vi "move_3.vi"(0 "Enum 3":enum16{"1", "2", "3", "4", "5"}(ring), 1 "Array 3":i32[](array[numeric]), 2 "Array 6":i32[](array[numeric]), 4 "Array in":i32[](array[numeric])) -> (5 "Array out":i32[](array[numeric]), 6 "Enum":T2(ring), 7 "Enum 2":T1(ring), 8 "Array 5":i32[](array[numeric]), 9 "Array 4":i32[](array[numeric]))   [LabVIEW 2016]
uses:
  <vilib>/NXT/Block Support/NXT_OutputPort.ctl
  <vilib>/NXT/NXTIO Xnodes/NXTIONodeSubVIs/NXTStopMotors.vi
  <vilib>/NXT/NXTIO Xnodes/NXTIONodeSubVIs/NXTMotorRunDistance.vi
  <vilib>/NXT/NXTIO Xnodes/NXTIONodeSubVIs/LEGOMotorStatus.vi
  <vilib>/NXT/NXTIO Xnodes/NXTIONodeSubVIs/NXTMoveMotors.vi
  <vilib>/NXT/NXTIO Xnodes/NXTIONodeSubVIs/LEGOResetMotors.vi
  <vilib>/NXT/Subs/LVHSConnector.ctl
  <vilib>/NXT/NXTIO Xnodes/AddressXNode/NXTIOAddress.xnode
  <vilib>/NXT/NXTIO Xnodes/NXTIOXNode/NXTIO.xnode
  <vilib>/NXT/LegoClasses/BrickReference/BrickReference.lvclass
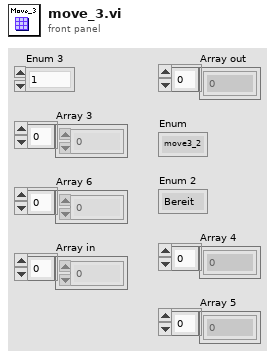
[diagram p1: front panel]
types:
  T1 = enum16{"Bereit", "Move 1", "Reference_pos", "Wait", "row1_check", "row2_check", "row3_check", "return", "move2", "move3", "move4", "move5", "end"}
  T2 = enum16{"move3_2", "move3_3", "move3_4", "move3_5"}
  T3 = enum16{"forward", "mark", "pause", "up", "return", "end"}
  T4 = typedef "NXT_OutputPort.ctl" = u8
  T5 = cluster{"Output Port":T4, "Output Port 2":T4, "Output Port 3":T4}
  T6 = enum16{"forward", "right", "mark", "pause", "up", "return", "end"}
  T7 = typedef "LVHSConnector.ctl" = refnum<class "BrickReference.lvclass">
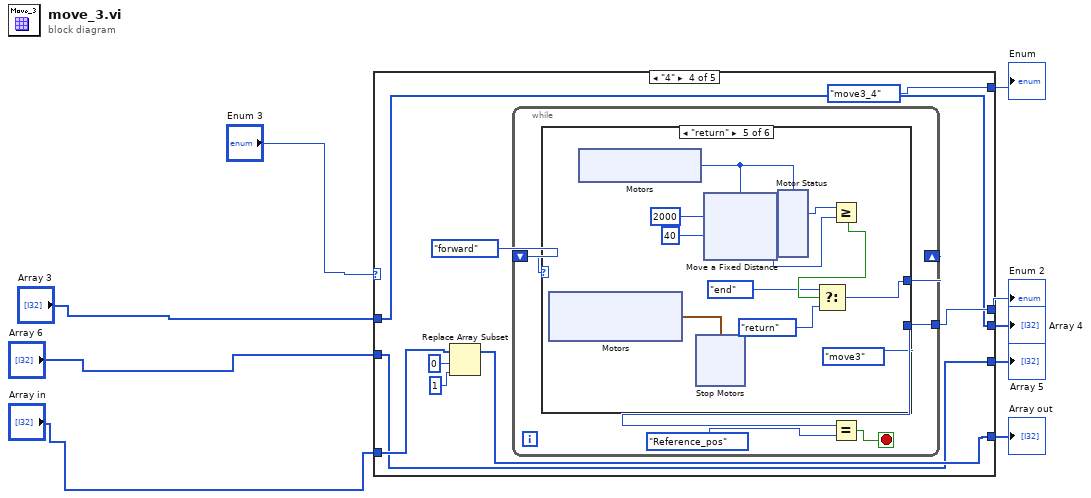
[diagram p0: block diagram]
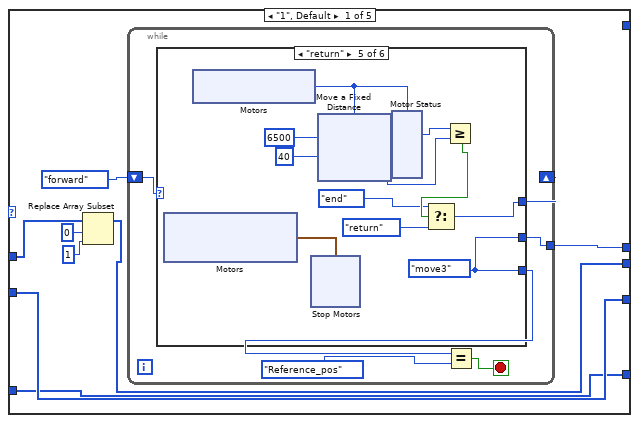
[diagram p2: hidden frame]
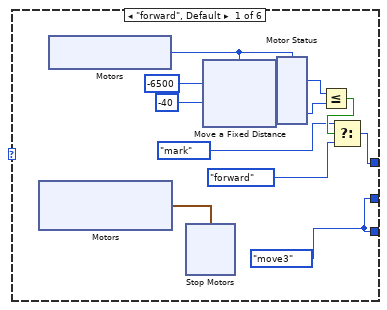
[diagram p3: hidden frame]
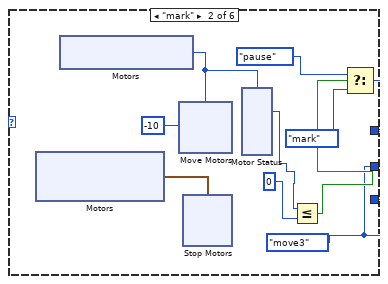
[diagram p4: hidden frame]
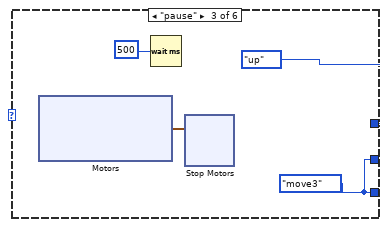
[diagram p5: hidden frame]
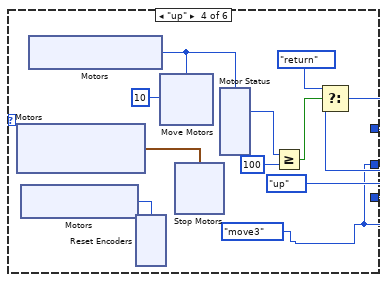
[diagram p6: hidden frame]
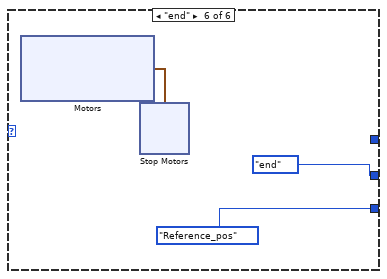
[diagram p7: hidden frame]
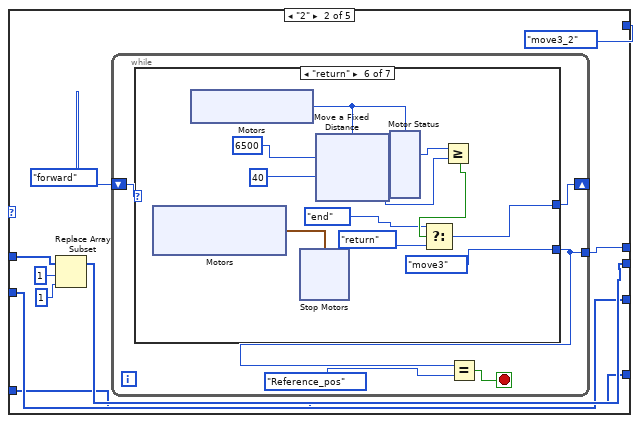
[diagram p8: hidden frame]
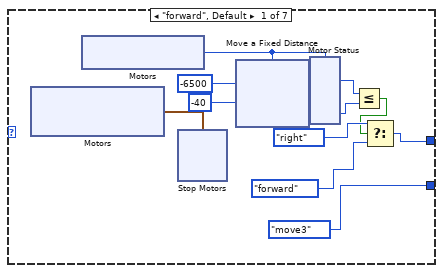
[diagram p9: hidden frame]
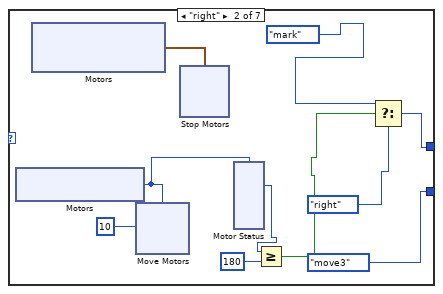
[diagram p10: hidden frame]
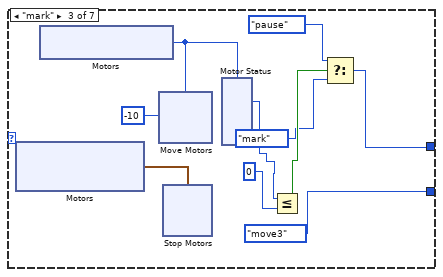
[diagram p11: hidden frame]
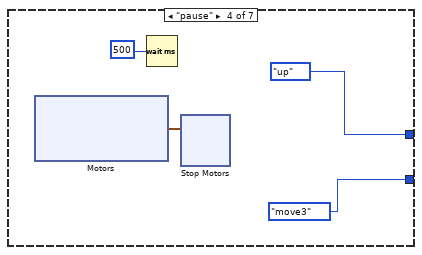
[diagram p12: hidden frame]
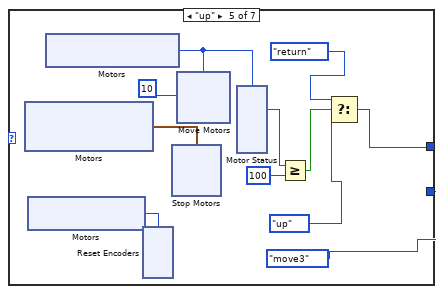
[diagram p13: hidden frame]
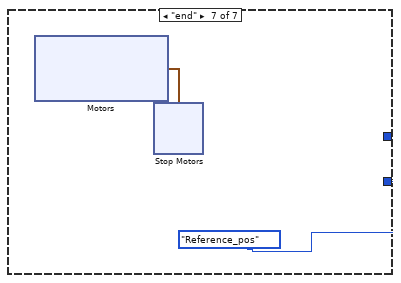
[diagram p14: hidden frame]
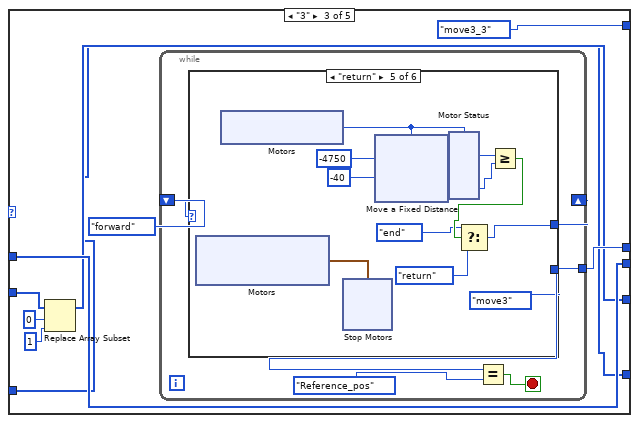
[diagram p15: hidden frame]
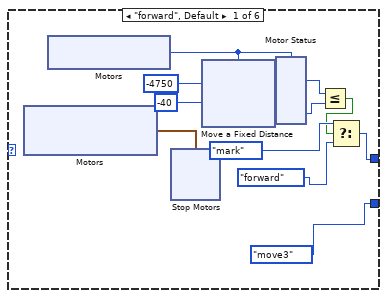
[diagram p16: hidden frame]
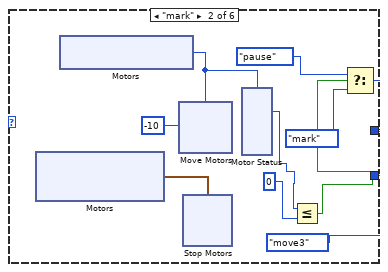
[diagram p17: hidden frame]
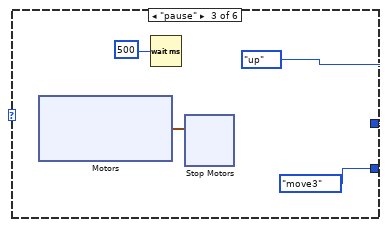
[diagram p18: hidden frame]
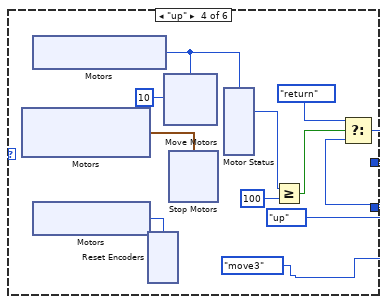
[diagram p19: hidden frame]
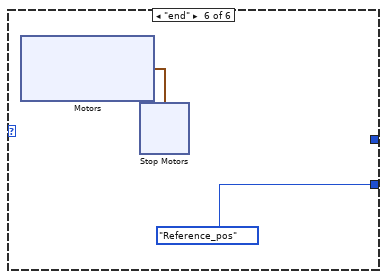
[diagram p20: hidden frame]
diagram:
  n1 = case shown="\"4\"" "Enum 3" {
    tunnel: [w16 w192 w398 w572 w745] -> w2
    tunnel: [_ T2."move3_2" T2."move3_3" T2."move3_4" T2."move3_5"] -> w3
    tunnel: "Array 6" -> [w15 w186 w393 w566 w738]
    tunnel: [w15 w186 w392 w566 w738] -> w5
    tunnel: [w10 w187 w396 w565 w739] -> w6
    tunnel: "Array 3" -> [w13 w188 w396 w565 w740]
    tunnel: [w14 w185 w391 w567 w741] -> w8
    tunnel: "Array in" -> [w14 w185 w391 w568 w741]
    frame "1", Default {
      n2 = Replace Array Subset(array=w13, new element=1 ("new element/subarray"), index=0) -> (w10:i32[])
      n3 = while {
        shift-right: [w23] -> _
        shift-left: T3."forward" -> [w22]
        tunnel: [w18] -> w16
        stop <- w20 stop-if-true
        n4 = case shown="\"return\"" w22 {
          tunnel: [w24 w67 T3."up" w109 w140 _] -> w23
          tunnel: [w33 w60 w92 w103 w149 T1."Reference_pos"] -> w21
          tunnel: [w33 w60 w92 w103 w149 T1."end"] -> w18
          frame "forward", Default {
            w28 = -6500 ("Distance 1")
            w33 = T1."move3"
            n5 = xnode "Motors"() -> ("Motor"=w34:cluster{"Port":T4, "Port":T4})
            n6 = xnode "Motors"() -> ("Motor"=w30:T4)
            n7 = xnode "Stop Motors"("Motors"=w34) -> ()  [unwired: 1 in, 1 out]
            n8 = xnode "Move a Fixed Distance"("Speed 1"=i8 -40, "Distance 1"=w28, "Motors"=w30) -> ("NXT/EV3"=w29:T7)  [unwired: 1 in]
            n9 = xnode "Motor Status"("Motors"=w30, "NXT/EV3"=w29) -> ("Position 1"=w31:i32)  [unwired: 2 out]
            n10 = Less Or Equal?(x=w31, y=w28) -> (x <= y?=w27:bool)
            n11 = Select(t=T3."mark", s=w27, f=T3."forward") -> (s? t:f=w24:T3)
          }
          frame "mark" {
            w60 = T1."move3"
            n12 = xnode "Motors"() -> ("Motor"=w69:cluster{"Port":T4, "Port":T4})
            n13 = xnode "Motors"() -> ("Motor"=w64:T4)
            n14 = xnode "Move Motors"("Power/Speed 1"=i8 -10, "Motors"=w64) -> ()  [unwired: 1 in, 1 out]
            n15 = xnode "Stop Motors"("Motors"=w69) -> ()  [unwired: 1 in, 1 out]
            n16 = xnode "Motor Status"("Motors"=w64) -> ("Position 1"=w63:i32)  [unwired: 1 in, 2 out]
            n17 = Less Or Equal?(x=w63, y=0) -> (x <= y?=w61:bool)
            n18 = Select(t=T3."pause", s=w61, f=T3."mark") -> (s? t:f=w67:T3)
          }
          frame "pause" {
            w92 = T1."move3"
            n19 = xnode "Motors"() -> ("Motor"=w95:cluster{"Port":T4, "Port":T4, "Port":T4})
            n20 = Wait (ms)(milliseconds to wait=u32 500 ("millisecond timer value")) -> ()  [unwired: 1 out]
            n21 = xnode "Stop Motors"("Motors"=w95) -> ()  [unwired: 1 in, 1 out]
          }
          frame "up" {
            w103 = T1."move3"
            n22 = xnode "Motors"() -> ("Motor"=w111:cluster{"Port":T4, "Port":T4})
            n23 = xnode "Motors"() -> ("Motor"=w102:T4)
            n24 = xnode "Motors"() -> ("Motor"=w105:T4)
            n25 = xnode "Reset Encoders"("Motors"=w102) -> ()  [unwired: 1 in, 1 out]
            n26 = xnode "Move Motors"("Power/Speed 1"=i8 10, "Motors"=w105) -> ()  [unwired: 1 in, 1 out]
            n27 = xnode "Stop Motors"("Motors"=w111) -> ()  [unwired: 1 in, 1 out]
            n28 = xnode "Motor Status"("Motors"=w105) -> ("Position 1"=w106:i32)  [unwired: 1 in, 2 out]
            n29 = Greater Or Equal?(x=w106, y=100) -> (x >= y?=w110:bool)
            n30 = Select(t=T3."return", s=w110, f=T3."up") -> (s? t:f=w109:T3)
          }
          frame "return" {
            w144 = 6500 ("Distance 1")
            w149 = T1."move3"
            n31 = xnode "Motors"() -> ("Motor"=w150:cluster{"Port":T4, "Port":T4})
            n32 = xnode "Motors"() -> ("Motor"=w147:T4)
            n33 = xnode "Stop Motors"("Motors"=w150) -> ()  [unwired: 1 in, 1 out]
            n34 = xnode "Move a Fixed Distance"("Speed 1"=i8 40, "Distance 1"=w144, "Motors"=w147) -> ("NXT/EV3"=w146:T7)  [unwired: 1 in]
            n35 = xnode "Motor Status"("Motors"=w147, "NXT/EV3"=w146) -> ("Position 1"=w145:i32)  [unwired: 2 out]
            n36 = Greater Or Equal?(x=w145, y=w144) -> (x >= y?=w143:bool)
            n37 = Select(t=T3."end", s=w143, f=T3."return") -> (s? t:f=w140:T3)
          }
          frame "end" {
            n38 = xnode "Motors"() -> ("Motor"=w178:cluster{"Port":T4, "Port":T4, "Port":T4})
            n39 = xnode "Stop Motors"("Motors"=w178) -> ()  [unwired: 1 in, 1 out]
          }
        }
        n40 = Equal?(x=w21, y=T1."Reference_pos") -> (x = y?=w20:bool)
      }
    }
    frame "2" {
      n41 = Replace Array Subset(array=w188, new element=1 ("new element/subarray"), index=1) -> (w187:i32[])
      n42 = while {
        shift-right: [w194] -> _
        shift-left: T6."forward" -> [w195]
        tunnel: [w198] -> w192
        stop <- w197 stop-if-true
        n43 = case shown="\"return\"" w195 {
          tunnel: [w200 w236 w268 T6."up" w310 w347 _] -> w194
          tunnel: [T1."move3" T1."move3" T1."move3" T1."move3" T1."move3" T1."move3" T1."Reference_pos"] -> w198
          frame "forward", Default {
            w203 = -6500 ("Distance 1")
            n44 = xnode "Motors"() -> ("Motor"=w209:cluster{"Port":T4, "Port":T4})
            n45 = xnode "Motors"() -> ("Motor"=w205:T4)
            n46 = xnode "Stop Motors"("Motors"=w209) -> ()  [unwired: 1 in, 1 out]
            n47 = xnode "Move a Fixed Distance"("Speed 1"=i8 -40, "Distance 1"=w203, "Motors"=w205) -> ("NXT/EV3"=w204:T7)  [unwired: 1 in]
            n48 = xnode "Motor Status"("Motors"=w205, "NXT/EV3"=w204) -> ("Position 1"=w206:i32)  [unwired: 2 out]
            n49 = Less Or Equal?(x=w206, y=w203) -> (x <= y?=w199:bool)
            n50 = Select(t=T6."right", s=w199, f=T6."forward") -> (s? t:f=w200:T6)
          }
          frame "right" {
            n51 = xnode "Motors"() -> ("Motor"=w244:T4)
            n52 = xnode "Motors"() -> ("Motor"=w243:cluster{"Port":T4, "Port":T4})
            n53 = xnode "Move Motors"("Power/Speed 1"=i8 10, "Motors"=w244) -> ()  [unwired: 1 in, 1 out]
            n54 = xnode "Stop Motors"("Motors"=w243) -> ()  [unwired: 1 in, 1 out]
            n55 = xnode "Motor Status"("Motors"=w244) -> ("Position 1"=w241:i32)  [unwired: 1 in, 2 out]
            n56 = Greater Or Equal?(x=w241, y=180) -> (x >= y?=w240:bool)
            n57 = Select(t=T6."mark", s=w240, f=T6."right") -> (s? t:f=w236:T6)
          }
          frame "mark" {
            n58 = xnode "Motors"() -> ("Motor"=w276:cluster{"Port":T4, "Port":T4})
            n59 = xnode "Motors"() -> ("Motor"=w274:T4)
            n60 = xnode "Move Motors"("Power/Speed 1"=i8 -10, "Motors"=w274) -> ()  [unwired: 1 in, 1 out]
            n61 = xnode "Stop Motors"("Motors"=w276) -> ()  [unwired: 1 in, 1 out]
            n62 = xnode "Motor Status"("Motors"=w274) -> ("Position 1"=w273:i32)  [unwired: 1 in, 2 out]
            n63 = Less Or Equal?(x=w273, y=0) -> (x <= y?=w271:bool)
            n64 = Select(t=T6."pause", s=w271, f=T6."mark") -> (s? t:f=w268:T6)
          }
          frame "pause" {
            n65 = xnode "Motors"() -> ("Motor"=w302:cluster{"Port":T4, "Port":T4, "Port":T4})
            n66 = Wait (ms)(milliseconds to wait=u32 500 ("millisecond timer value")) -> ()  [unwired: 1 out]
            n67 = xnode "Stop Motors"("Motors"=w302) -> ()  [unwired: 1 in, 1 out]
          }
          frame "up" {
            n68 = xnode "Motors"() -> ("Motor"=w317:cluster{"Port":T4, "Port":T4})
            n69 = xnode "Motors"() -> ("Motor"=w309:T4)
            n70 = xnode "Motors"() -> ("Motor"=w314:T4)
            n71 = xnode "Reset Encoders"("Motors"=w309) -> ()  [unwired: 1 in, 1 out]
            n72 = xnode "Stop Motors"("Motors"=w317) -> ()  [unwired: 1 in, 1 out]
            n73 = xnode "Move Motors"("Power/Speed 1"=i8 10, "Motors"=w314) -> ()  [unwired: 1 in, 1 out]
            n74 = xnode "Motor Status"("Motors"=w314) -> ("Position 1"=w315:i32)  [unwired: 1 in, 2 out]
            n75 = Greater Or Equal?(x=w315, y=100) -> (x >= y?=w316:bool)
            n76 = Select(t=T6."return", s=w316, f=T6."up") -> (s? t:f=w310:T6)
          }
          frame "return" {
            w351 = 6500 ("Distance 1")
            n77 = xnode "Motors"() -> ("Motor"=w356:cluster{"Port":T4, "Port":T4})
            n78 = xnode "Motors"() -> ("Motor"=w355:T4)
            n79 = xnode "Stop Motors"("Motors"=w356) -> ()  [unwired: 1 in, 1 out]
            n80 = xnode "Move a Fixed Distance"("Speed 1"=i8 40, "Distance 1"=w351, "Motors"=w355) -> ("NXT/EV3"=w354:T7)  [unwired: 1 in]
            n81 = xnode "Motor Status"("Motors"=w355, "NXT/EV3"=w354) -> ("Position 1"=w353:i32)  [unwired: 2 out]
            n82 = Greater Or Equal?(x=w353, y=w351) -> (x >= y?=w352:bool)
            n83 = Select(t=T6."end", s=w352, f=T6."return") -> (s? t:f=w347:T6)
          }
          frame "end" {
            n84 = xnode "Motors"() -> ("Motor"=w383:cluster{"Port":T4, "Port":T4, "Port":T4})
            n85 = xnode "Stop Motors"("Motors"=w383) -> ()  [unwired: 1 in, 1 out]
          }
        }
        n86 = Equal?(x=w198, y=T1."Reference_pos") -> (x = y?=w197:bool)
      }
    }
    frame "3" {
      n87 = Replace Array Subset(array=w393, new element=1 ("new element/subarray"), index=0) -> (w392:i32[])
      n88 = while {
        shift-right: [w404] -> _
        shift-left: T3."forward" -> [w403]
        tunnel: [w402] -> w398
        stop <- w401 stop-if-true
        n89 = case shown="\"return\"" w403 {
          tunnel: [w405 w448 T3."up" w490 w521 _] -> w404
          tunnel: [T1."move3" T1."move3" T1."move3" T1."move3" T1."move3" T1."Reference_pos"] -> w402
          frame "forward", Default {
            w409 = -4750 ("Distance 1")
            n90 = xnode "Motors"() -> ("Motor"=w415:cluster{"Port":T4, "Port":T4})
            n91 = xnode "Motors"() -> ("Motor"=w411:T4)
            n92 = xnode "Stop Motors"("Motors"=w415) -> ()  [unwired: 1 in, 1 out]
            n93 = xnode "Move a Fixed Distance"("Speed 1"=i8 -40, "Distance 1"=w409, "Motors"=w411) -> ("NXT/EV3"=w410:T7)  [unwired: 1 in]
            n94 = xnode "Motor Status"("Motors"=w411, "NXT/EV3"=w410) -> ("Position 1"=w412:i32)  [unwired: 2 out]
            n95 = Less Or Equal?(x=w412, y=w409) -> (x <= y?=w406:bool)
            n96 = Select(t=T3."mark", s=w406, f=T3."forward") -> (s? t:f=w405:T3)
          }
          frame "mark" {
            n97 = xnode "Motors"() -> ("Motor"=w450:cluster{"Port":T4, "Port":T4})
            n98 = xnode "Motors"() -> ("Motor"=w445:T4)
            n99 = xnode "Move Motors"("Power/Speed 1"=i8 -10, "Motors"=w445) -> ()  [unwired: 1 in, 1 out]
            n100 = xnode "Stop Motors"("Motors"=w450) -> ()  [unwired: 1 in, 1 out]
            n101 = xnode "Motor Status"("Motors"=w445) -> ("Position 1"=w444:i32)  [unwired: 1 in, 2 out]
            n102 = Less Or Equal?(x=w444, y=0) -> (x <= y?=w442:bool)
            n103 = Select(t=T3."pause", s=w442, f=T3."mark") -> (s? t:f=w448:T3)
          }
          frame "pause" {
            n104 = xnode "Motors"() -> ("Motor"=w476:cluster{"Port":T4, "Port":T4, "Port":T4})
            n105 = Wait (ms)(milliseconds to wait=u32 500 ("millisecond timer value")) -> ()  [unwired: 1 out]
            n106 = xnode "Stop Motors"("Motors"=w476) -> ()  [unwired: 1 in, 1 out]
          }
          frame "up" {
            n107 = xnode "Motors"() -> ("Motor"=w492:cluster{"Port":T4, "Port":T4})
            n108 = xnode "Motors"() -> ("Motor"=w486:T4)
            n109 = xnode "Motors"() -> ("Motor"=w483:T4)
            n110 = xnode "Reset Encoders"("Motors"=w483) -> ()  [unwired: 1 in, 1 out]
            n111 = xnode "Move Motors"("Power/Speed 1"=i8 10, "Motors"=w486) -> ()  [unwired: 1 in, 1 out]
            n112 = xnode "Stop Motors"("Motors"=w492) -> ()  [unwired: 1 in, 1 out]
            n113 = xnode "Motor Status"("Motors"=w486) -> ("Position 1"=w487:i32)  [unwired: 1 in, 2 out]
            n114 = Greater Or Equal?(x=w487, y=100) -> (x >= y?=w491:bool)
            n115 = Select(t=T3."return", s=w491, f=T3."up") -> (s? t:f=w490:T3)
          }
          frame "return" {
            w525 = -4750 ("Distance 1")
            n116 = xnode "Motors"() -> ("Motor"=w531:cluster{"Port":T4, "Port":T4})
            n117 = xnode "Motors"() -> ("Motor"=w528:T4)
            n118 = xnode "Stop Motors"("Motors"=w531) -> ()  [unwired: 1 in, 1 out]
            n119 = xnode "Move a Fixed Distance"("Speed 1"=i8 -40, "Distance 1"=w525, "Motors"=w528) -> ("NXT/EV3"=w527:T7)  [unwired: 1 in]
            n120 = xnode "Motor Status"("Motors"=w528, "NXT/EV3"=w527) -> ("Position 1"=w526:i32)  [unwired: 2 out]
            n121 = Greater Or Equal?(x=w526, y=w525) -> (x >= y?=w524:bool)
            n122 = Select(t=T3."end", s=w524, f=T3."return") -> (s? t:f=w521:T3)
          }
          frame "end" {
            n123 = xnode "Motors"() -> ("Motor"=w558:cluster{"Port":T4, "Port":T4, "Port":T4})
            n124 = xnode "Stop Motors"("Motors"=w558) -> ()  [unwired: 1 in, 1 out]
          }
        }
        n125 = Equal?(x=w402, y=T1."Reference_pos") -> (x = y?=w401:bool)
      }
    }
    frame "4" {
      n126 = Replace Array Subset(array=w568, new element=1 ("new element/subarray"), index=0) -> (w567:i32[])
      n127 = while {
        shift-right: [w578] -> _
        shift-left: T3."forward" -> [w577]
        tunnel: [w576] -> w572
        stop <- w575 stop-if-true
        n128 = case shown="\"return\"" w577 {
          tunnel: [w580 w622 w647 w663 w695 _] -> w578
          tunnel: [T1."move3" T1."move3" T1."move3" T1."move3" T1."move3" T1."Reference_pos"] -> w576
          frame "forward", Default {
            w583 = -3000 ("Distance 1")
            n129 = xnode "Motors"() -> ("Motor"=w585:T4)
            n130 = xnode "Motors"() -> ("Motor"=w589:cluster{"Port":T4, "Port":T4})
            n131 = xnode "Stop Motors"("Motors"=w589) -> ()  [unwired: 1 in, 1 out]
            n132 = xnode "Move a Fixed Distance"("Speed 1"=i8 -40, "Distance 1"=w583, "Motors"=w585) -> ("NXT/EV3"=w584:T7)  [unwired: 1 in]
            n133 = xnode "Motor Status"("Motors"=w585, "NXT/EV3"=w584) -> ("Position 1"=w586:i32)  [unwired: 2 out]
            n134 = Less Or Equal?(x=w586, y=w583) -> (x <= y?=w579:bool)
            n135 = Select(t=T3."mark", s=w579, f=T3."forward") -> (s? t:f=w580:T3)
          }
          frame "mark" {
            n136 = xnode "Motors"() -> ("Motor"=w624:cluster{"Port":T4, "Port":T4})
            n137 = xnode "Motors"() -> ("Motor"=w619:T4)
            n138 = xnode "Move Motors"("Power/Speed 1"=i8 -10, "Motors"=w619) -> ()  [unwired: 1 in, 1 out]
            n139 = xnode "Stop Motors"("Motors"=w624) -> ()  [unwired: 1 in, 1 out]
            n140 = xnode "Motor Status"("Motors"=w619) -> ("Position 1"=w618:i32)  [unwired: 1 in, 2 out]
            n141 = Less Or Equal?(x=w618, y=0) -> (x <= y?=w616:bool)
            n142 = Select(t=T3."pause", s=w616, f=T3."mark") -> (s? t:f=w622:T3)
          }
          frame "pause" {
            n143 = xnode "Motors"() -> ("Motor"=w648:cluster{"Port":T4, "Port":T4})
            n144 = call "x0_move2.vi"() -> ("Enum"=w647:T3)  [unwired: 1 in]
            n145 = xnode "Stop Motors"("Motors"=w648) -> ()  [unwired: 1 in, 1 out]
          }
          frame "up" {
            n146 = xnode "Motors"() -> ("Motor"=w665:cluster{"Port":T4, "Port":T4})
            n147 = xnode "Motors"() -> ("Motor"=w656:T4)
            n148 = xnode "Motors"() -> ("Motor"=w659:T4)
            n149 = xnode "Reset Encoders"("Motors"=w656) -> ()  [unwired: 1 in, 1 out]
            n150 = xnode "Stop Motors"("Motors"=w665) -> ()  [unwired: 1 in, 1 out]
            n151 = xnode "Move Motors"("Power/Speed 1"=i8 10, "Motors"=w659) -> ()  [unwired: 1 in, 1 out]
            n152 = xnode "Motor Status"("Motors"=w659) -> ("Position 1"=w660:i32)  [unwired: 1 in, 2 out]
            n153 = Greater Or Equal?(x=w660, y=100) -> (x >= y?=w664:bool)
            n154 = Select(t=T3."return", s=w664, f=T3."up") -> (s? t:f=w663:T3)
          }
          frame "return" {
            w694 = 2000 ("Distance 1")
            n155 = xnode "Motors"() -> ("Motor"=w704:cluster{"Port":T4, "Port":T4})
            n156 = xnode "Motors"() -> ("Motor"=w701:T4)
            n157 = xnode "Stop Motors"("Motors"=w704) -> ()  [unwired: 1 in, 1 out]
            n158 = xnode "Move a Fixed Distance"("Speed 1"=i8 40, "Distance 1"=w694, "Motors"=w701) -> ("NXT/EV3"=w700:T7)  [unwired: 1 in]
            n159 = xnode "Motor Status"("Motors"=w701, "NXT/EV3"=w700) -> ("Position 1"=w699:i32)  [unwired: 2 out]
            n160 = Greater Or Equal?(x=w699, y=w694) -> (x >= y?=w698:bool)
            n161 = Select(t=T3."end", s=w698, f=T3."return") -> (s? t:f=w695:T3)
          }
          frame "end" {
            n162 = xnode "Motors"() -> ("Motor"=w731:cluster{"Port":T4, "Port":T4, "Port":T4})
            n163 = xnode "Stop Motors"("Motors"=w731) -> ()  [unwired: 1 in, 1 out]
          }
        }
        n164 = Equal?(x=w576, y=T1."Reference_pos") -> (x = y?=w575:bool)
      }
    }
    frame "5" {
      n165 = Replace Array Subset(array=w740, new element=1 ("new element/subarray"), index=2) -> (w739:i32[])
      n166 = while {
        shift-right: [w747] -> _
        shift-left: T6."forward" -> [w748]
        tunnel: [w751] -> w745
        stop <- w750 stop-if-true
        n167 = case shown="\"return\"" w748 {
          tunnel: [w754 w789 w821 T6."up" w863 w900 _] -> w747
          tunnel: [T1."move3" T1."move3" T1."move3" T1."move3" T1."move3" T1."move3" T1."Reference_pos"] -> w751
          frame "forward", Default {
            w756 = -6500 ("Distance 1")
            n168 = xnode "Motors"() -> ("Motor"=w758:T4)
            n169 = xnode "Motors"() -> ("Motor"=w762:cluster{"Port":T4, "Port":T4})
            n170 = xnode "Move a Fixed Distance"("Speed 1"=i8 -40, "Distance 1"=w756, "Motors"=w758) -> ("NXT/EV3"=w757:T7)  [unwired: 1 in]
            n171 = xnode "Stop Motors"("Motors"=w762) -> ()  [unwired: 1 in, 1 out]
            n172 = xnode "Motor Status"("Motors"=w758, "NXT/EV3"=w757) -> ("Position 1"=w759:i32)  [unwired: 2 out]
            n173 = Less Or Equal?(x=w759, y=w756) -> (x <= y?=w755:bool)
            n174 = Select(t=T6."right", s=w755, f=T6."forward") -> (s? t:f=w754:T6)
          }
          frame "right" {
            n175 = xnode "Motors"() -> ("Motor"=w797:T4)
            n176 = xnode "Motors"() -> ("Motor"=w796:cluster{"Port":T4, "Port":T4})
            n177 = xnode "Move Motors"("Power/Speed 1"=i8 10, "Motors"=w797) -> ()  [unwired: 1 in, 1 out]
            n178 = xnode "Stop Motors"("Motors"=w796) -> ()  [unwired: 1 in, 1 out]
            n179 = xnode "Motor Status"("Motors"=w797) -> ("Position 1"=w794:i32)  [unwired: 1 in, 2 out]
            n180 = Greater Or Equal?(x=w794, y=360) -> (x >= y?=w793:bool)
            n181 = Select(t=T6."mark", s=w793, f=T6."right") -> (s? t:f=w789:T6)
          }
          frame "mark" {
            n182 = xnode "Motors"() -> ("Motor"=w829:cluster{"Port":T4, "Port":T4})
            n183 = xnode "Motors"() -> ("Motor"=w827:T4)
            n184 = xnode "Move Motors"("Power/Speed 1"=i8 -10, "Motors"=w827) -> ()  [unwired: 1 in, 1 out]
            n185 = xnode "Stop Motors"("Motors"=w829) -> ()  [unwired: 1 in, 1 out]
            n186 = xnode "Motor Status"("Motors"=w827) -> ("Position 1"=w826:i32)  [unwired: 1 in, 2 out]
            n187 = Less Or Equal?(x=w826, y=0) -> (x <= y?=w824:bool)
            n188 = Select(t=T6."pause", s=w824, f=T6."mark") -> (s? t:f=w821:T6)
          }
          frame "pause" {
            n189 = xnode "Motors"() -> ("Motor"=w855:cluster{"Port":T4, "Port":T4, "Port":T4})
            n190 = Wait (ms)(milliseconds to wait=u32 500 ("millisecond timer value")) -> ()  [unwired: 1 out]
            n191 = xnode "Stop Motors"("Motors"=w855) -> ()  [unwired: 1 in, 1 out]
          }
          frame "up" {
            n192 = xnode "Motors"() -> ("Motor"=w862:T4)
            n193 = xnode "Motors"() -> ("Motor"=w870:cluster{"Port":T4, "Port":T4})
            n194 = xnode "Motors"() -> ("Motor"=w867:T4)
            n195 = xnode "Reset Encoders"("Motors"=w862) -> ()  [unwired: 1 in, 1 out]
            n196 = xnode "Move Motors"("Power/Speed 1"=i8 10, "Motors"=w867) -> ()  [unwired: 1 in, 1 out]
            n197 = xnode "Stop Motors"("Motors"=w870) -> ()  [unwired: 1 in, 1 out]
            n198 = xnode "Motor Status"("Motors"=w867) -> ("Position 1"=w868:i32)  [unwired: 1 in, 2 out]
            n199 = Greater Or Equal?(x=w868, y=100) -> (x >= y?=w869:bool)
            n200 = Select(t=T6."return", s=w869, f=T6."up") -> (s? t:f=w863:T6)
          }
          frame "return" {
            w904 = 6500 ("Distance 1")
            n201 = xnode "Motors"() -> ("Motor"=w909:cluster{"Port":T4, "Port":T4})
            n202 = xnode "Motors"() -> ("Motor"=w907:T4)
            n203 = xnode "Stop Motors"("Motors"=w909) -> ()  [unwired: 1 in, 1 out]
            n204 = xnode "Move a Fixed Distance"("Speed 1"=i8 40, "Distance 1"=w904, "Motors"=w907) -> ("NXT/EV3"=w906:T7)  [unwired: 1 in]
            n205 = xnode "Motor Status"("Motors"=w907, "NXT/EV3"=w906) -> ("Position 1"=w905:i32)  [unwired: 2 out]
            n206 = Greater Or Equal?(x=w905, y=w904) -> (x >= y?=w901:bool)
            n207 = Select(t=T6."end", s=w901, f=T6."return") -> (s? t:f=w900:T6)
          }
          frame "end" {
            n208 = xnode "Motors"() -> ("Motor"=w936:cluster{"Port":T4, "Port":T4, "Port":T4})
            n209 = xnode "Stop Motors"("Motors"=w936) -> ()  [unwired: 1 in, 1 out]
          }
        }
        n210 = Equal?(x=w751, y=T1."Reference_pos") -> (x = y?=w750:bool)
      }
    }
  }
  "Array out" <- w8
  "Array 4" <- w6
  "Array 5" <- w5
  "Enum" <- w3
  "Enum 2" <- w2
